vi "Base64url_Encode.vi"(7 "Padded (T)":bool=TRUE, 10 "error in (no error)":errorcluster, 11 "String":string) -> (2 "error out":errorcluster, 3 "Encoded String":string)   [LabVIEW 2017, in "Serializer.Base64.lvclass"]
doc: "<B>Base 64 Encoding with URL and Filename Safe Alphabet</B>\n\n Provides Base 64 encoding with a URL and filename safe alphabet.\n\n The pad character \"=\" is typically percent-encoded when used in an\n URI, but if the data length is known implicitly, this can be\n avoided by skipping the padding.\n\n Base64url encoding is technically identical to the Base64, except\n for the 62:nd and 63:rd alphabet characters and the optional padding.\n\n This encoding may be referred to as \"base64url\". This encoding\n should not be regarded as the same as the \"base64\" encoding and\n should NOT be referred to as only \"base64\"."
uses:
  Serializer.Base64.lvclass
  Serializer.Base64.lvclass/Serializer.Base64.ctl
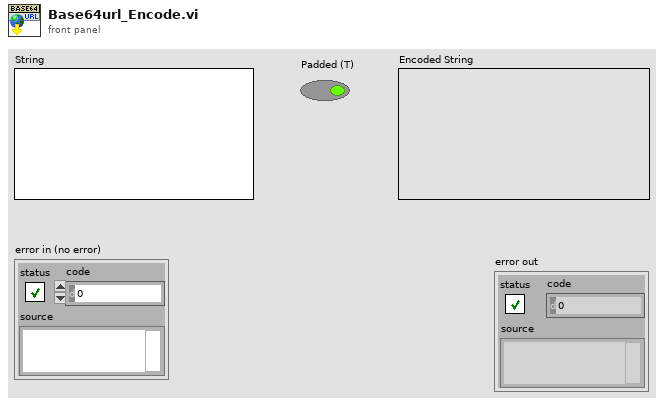
[diagram p1: front panel]
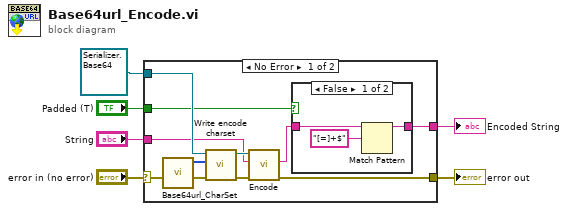
[diagram p0: block diagram]
diagram:
  n1 = case shown="No Error" "error in (no error)" {
    selector: "error in (no error)" -> [w14 w21]
    tunnel: "String" -> [w12 _]
    tunnel: [w10 w21] -> w4
    tunnel: refnum<class "Serializer.Base64.lvclass"> refnum ("Serializer.Base64 in") -> [w15 _]
    tunnel: [w7 _] -> w2
    tunnel: "Padded (T)" -> [w9 _]
    frame No Error {
      n2 = call "Base64url_CharSet.vi"() -> ("base64 URL charset"=w16:u8[])  [unwired: 11 in]
      n3 = call "Write encode charset.vi"("error in (no error)"=w14, "encode charset"=w16, "Serializer.Base64 in"=w15) -> ("error out"=w11:errorcluster, "Serializer.Base64 out"=w13:refnum<class "Serializer.Base64.lvclass">)  [unwired: 7 in]
      n4 = call "Encode.vi"("error in (no error)"=w11, "String"=w12, "Serializer.Base64 in"=w13) -> ("error out"=w10:errorcluster, "encoded string"=w8:string)  [unwired: 6 in, 1 out]
      n5 = case shown="False" w9 {
        tunnel: w8 -> [w19 w20]
        tunnel: [w17 w20] -> w7
        frame False {
          n6 = Match Pattern(string=w19, regular expression="[=]+$") -> (before substring=w17:string)  [unwired: 1 in, 3 out]
        }
        frame True {
        }
      }
    }
    frame Error {
    }
  }
  "Encoded String" <- w2
  "error out" <- w4
